vi "ExcimSavePanel.vi"(8 "error in":errorcluster) -> (0 "error out":errorcluster, 3 "Chaîne":string)   [LabVIEW 2010, in "PhotoLum.lvclass"]
uses:
  PhotoLum.lvclass
panel:
  in  "RepRate":i32=5 caption="Taux Répétition(PPS)" min=0 step=1
  in  "OtherMat":string caption="Matériaux (autres)"
  in  "Matériaux":u16(ring) items=["AlGaAs", "AlN", "AlP", "GaAs", "GaN", "Ge", "InP", "Si", "SiGe", "Autres"]
  in  "unit":u16(ring) caption="Unités\nPre-amp." items=["mA/V", "µA/V", "nA/V", "pA/V"]
  in  "Facteur":u16(ring) caption="Facteur Pre-amp." items=["1", "2", "5", "10", "20", "50", "100", "200", "500"]
  in  "Preamp":u16(ring) caption="Pre-amplificateur" items=["Aucun", "SR570 Current Preamp", "SR560 Voltage Preamp"]
  in  "PLaser":dbl=1000.0 caption="Énergie Laser(mJ)" min=0.0 step=0.1 format="%#.1f"
  in  "Temp":dbl=293.0 caption="Température(°K)" min=0.0 step=0.1 format="%#.1f"
  in  "Annuler":bool
  in  "Save":bool
  in  "Autres":string
  in  "Filtre":u16(ring) caption="Filtre Entrée" items=["Aucun", "CGA 225", "Mauve", "Jaune 495nm", "Vert", "Orange", "Rouge 665nm", "Rouge 850nm", "SI"]
  in  "LN Cooled":bool
  in  "Échantillon":string
  in  "Détecteur":u16(ring) items=["Oriel 70680 with R928"]
  in  "Réseaux":u16(ring) items=["Oriel 33010FL01-080R (400nm)", "Oriel 77234 (1um)"]
  in  "2xInput":bool
  in  "OutputSlit":dbl caption="Largeur de fente de sortie (mm)"
  in  "InputSlit":dbl caption="Largeur de fente d'entrée (mm)"
  # "Paramètres du balayage"
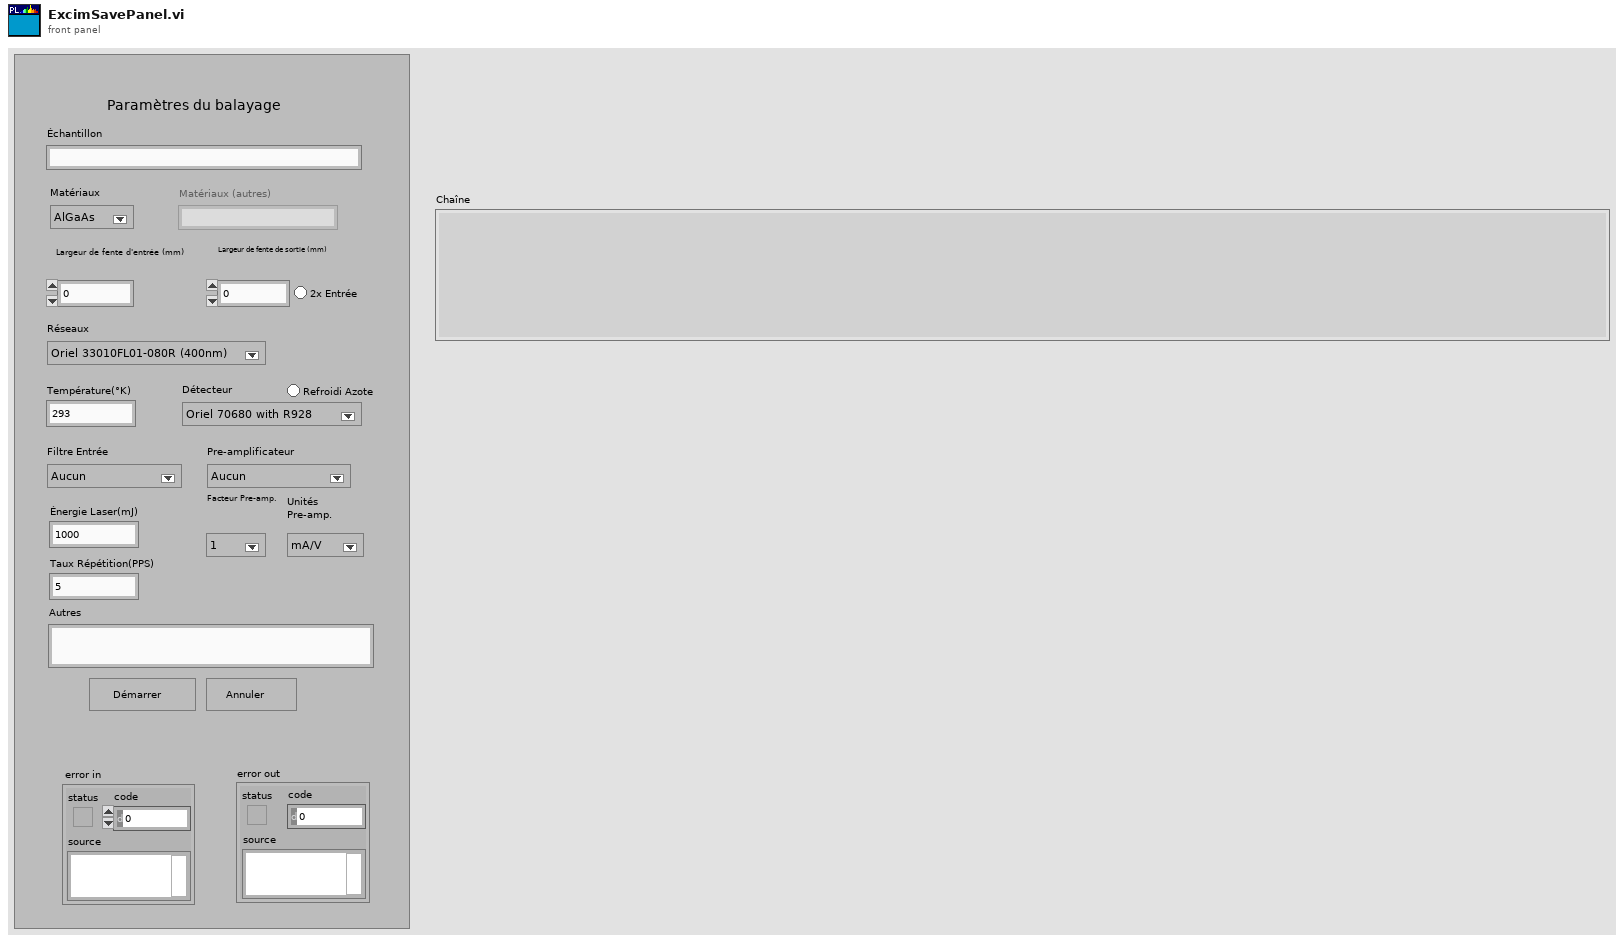
[diagram p1: front panel]
types:
  T1 = enum8{"Enabled", "Disabled", "Disabled and Grayed Out"}
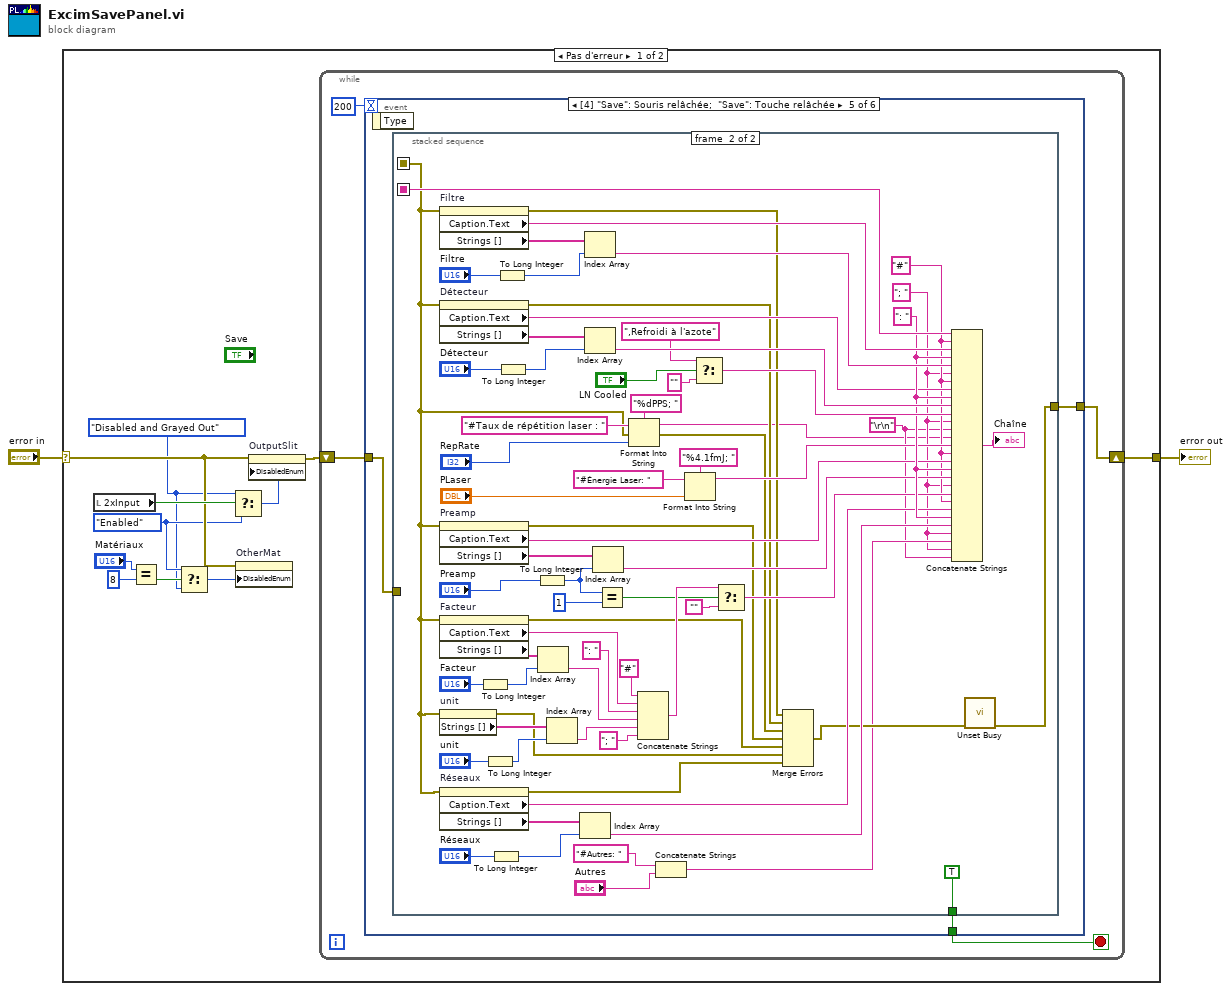
[diagram p0: block diagram]
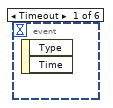
[diagram p2: hidden frame]
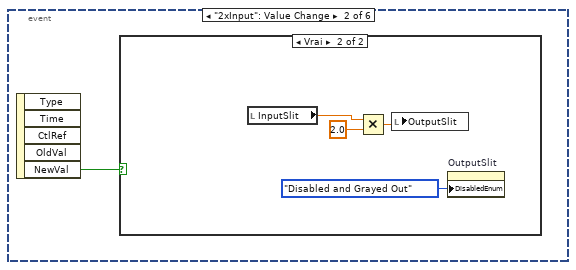
[diagram p3: hidden frame]
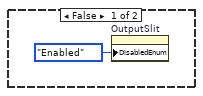
[diagram p4: hidden frame]
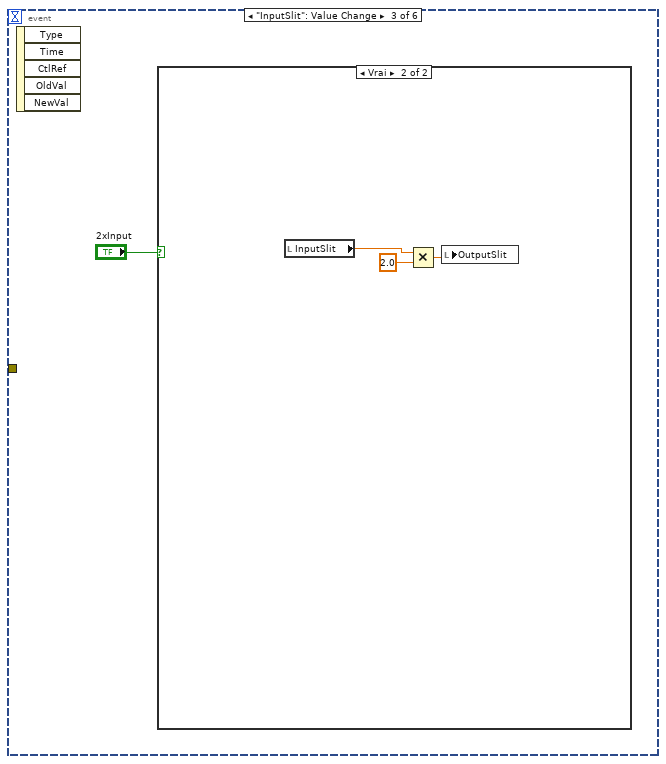
[diagram p5: hidden frame]
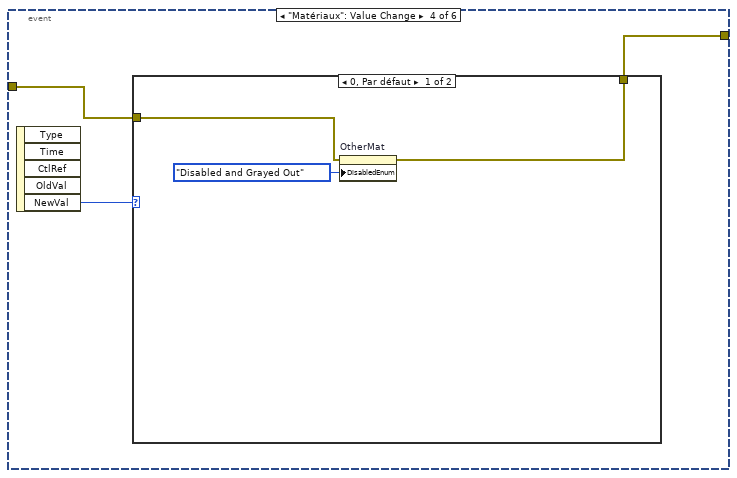
[diagram p7: hidden frame]
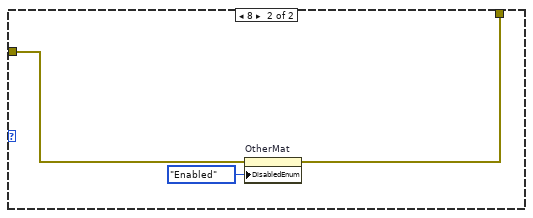
[diagram p8: hidden frame]
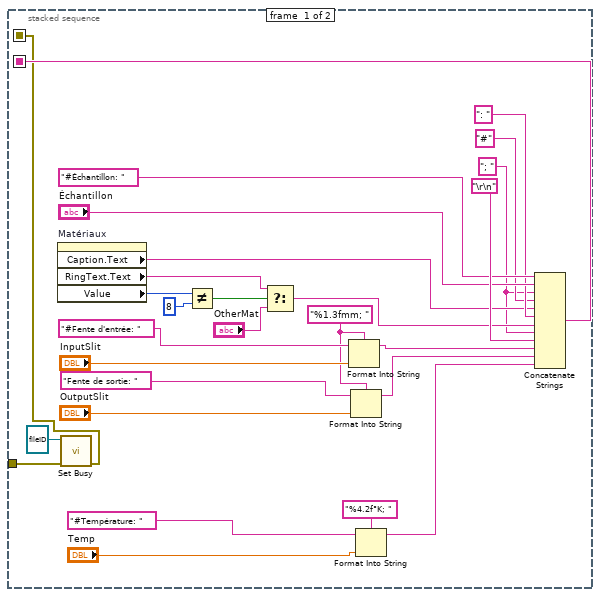
[diagram p9: hidden frame]
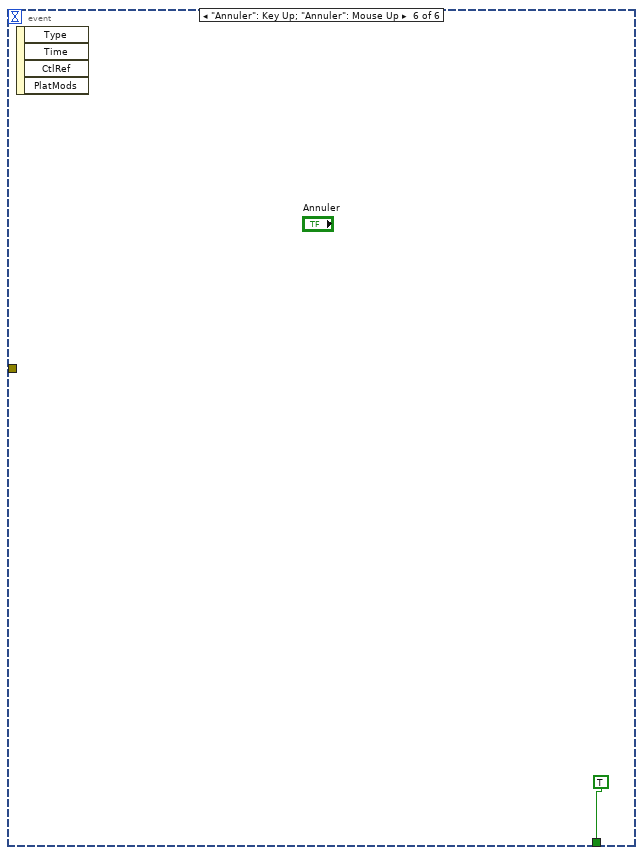
[diagram p10: hidden frame]
diagram:
  n1 = case shown="Pas d'erreur" "error in" {
    selector: "error in" -> [w9 w138]
    tunnel: [w13 w138] -> w2
    frame No Error {
      w4 = T1."Disabled and Grayed Out" ("Désactivé")
      w5 = T1."Enabled" ("Désactivé")
      n2 = local read "2xInput"() -> (w11:bool)
      n3 = Equal?(x="Matériaux", y=u16 8) -> (x = y?=w6:bool)
      n4 = Select(t=w5, s=w6, f=w4) -> (s? t:f=w3:T1)
      n5 = Select(t=w4, s=w11, f=w5) -> (s? t:f=w10:T1)
      n6 = property on="OtherMat" class="Ch"(error in=w9, "DisabledEnum"=w3) -> ()  [unwired: 1 in, 2 out]
      n7 = property on="OutputSlit" class="NumDig (strict)"(error in=w9, "DisabledEnum"=w10) -> (error out=w12:errorcluster)  [unwired: 1 in, 1 out]
      n8 = while {
        shift-right: [w14] -> w13
        shift-left: w12 -> [w15]
        stop <- w16 stop-if-true
        n9 = event shown="[4] \"Save\": Souris relâchée;  \"Save\": Touche relâchée" {
          selector: _ -> [_ _ _ _ _ _]
          dyn-events: _ -> [_ _ _ _ _ _]
          timeout: 200 -> [_ _ _ _ _ _]
          tunnel: [_ _ _ _ w39 TRUE] -> w16
          tunnel: w15 -> [_ _ _ w29 w38 _]
          tunnel: [_ _ _ w28 w37 _] -> w14
          event Timeout {
            n10 = event-data() -> ()  [unwired: 1 in, 2 out]
          }
          event "2xInput": Value Change {
            n11 = event-data() -> ("NewVal"=w18:bool)  [unwired: 1 in, 4 out]
            n12 = case shown="Vrai" w18 {
              frame False {
                n13 = property on="OutputSlit" class="NumDig (strict)"("DisabledEnum"=T1."Enabled" ("Désactivé")) -> ()  [unwired: 2 in, 2 out]
              }
              frame True {
                n14 = local read "InputSlit"() -> (w20:dbl)
                n15 = Multiply(x=w20, y=2.0) -> (x*y=w22:dbl)
                n16 = local write "OutputSlit"(w22) -> ()
                n17 = property on="OutputSlit" class="NumDig (strict)"("DisabledEnum"=T1."Disabled and Grayed Out" ("Désactivé")) -> ()  [unwired: 2 in, 2 out]
              }
            }
          }
          event "InputSlit": Value Change {
            n18 = event-data() -> ()  [unwired: 1 in, 5 out]
            n19 = case shown="Vrai" "2xInput" {
              frame False {
              }
              frame True {
                n20 = local read "InputSlit"() -> (w25:dbl)
                n21 = Multiply(x=w25, y=2.0) -> (x*y=w27:dbl)
                n22 = local write "OutputSlit"(w27) -> ()
              }
            }
          }
          event "Matériaux": Value Change {
            n23 = event-data() -> ("NewVal"=w30:u16)  [unwired: 1 in, 4 out]
            n24 = case shown="0, Par défaut" w30 {
              tunnel: w29 -> [w32 w35]
              tunnel: [w31 w34] -> w28
              frame 0, Default {
                n25 = property on="OtherMat" class="Ch"(error in=w32, "DisabledEnum"=T1."Disabled and Grayed Out" ("Désactivé")) -> (error out=w31:errorcluster)  [unwired: 1 in, 1 out]
              }
              frame 8 {
                n26 = property on="OtherMat" class="Ch"(error in=w35, "DisabledEnum"=T1."Enabled" ("Désactivé")) -> (error out=w34:errorcluster)  [unwired: 1 in, 1 out]
              }
            }
          }
          event "Save": Mouse Up; "Save": Key Up {
            n27 = event-data() -> ()  [unwired: 1 in, 1 out]
            n28 = stacked-sequence {
              seq-local: [w51 _] -> [_ w120]
              seq-local: [w40 _] -> [_ w69]
              tunnel: [_ TRUE] -> w39
              tunnel: w38 -> [w53 _]
              tunnel: [_ w80] -> w37
              frame #0 {
                w58 = "%1.3fmm; " ("chaîne de format")
                w41 = "; " ("chaîne")
                n29 = property on="Matériaux" class="MDér (strict)"() -> ("Caption.Text"=w48:string, "RingText.Text"=w44:string, "Value"=w46:u16)  [unwired: 2 in, 2 out]
                n30 = call <vilib>:"Set Busy.vi"("error in (no error)"=w53, "cursor ID"=refnum<k1> refnum) -> ("error out"=w40:errorcluster)  [unwired: 8 in, 1 out]
                n31 = Not Equal?(x=w46, y=u16 8) -> (x != y?=w45:bool)
                n32 = Select(t=w44, s=w45, f="OtherMat") -> (s? t:f=w42:string)
                n33 = Format Into String(format string=w58, initial string="#Fente d'entrée: " ("chaîne"), "InputSlit") -> (resulting string=w62:string)  [unwired: 1 in, 1 out]
                n34 = Format Into String(format string=w58, initial string="Fente de sortie: " ("chaîne"), "OutputSlit") -> (resulting string=w61:string)  [unwired: 1 in, 1 out]
                n35 = Format Into String(format string="%4.2f°K; " ("chaîne de format"), initial string="#Température: " ("string"), "Temp") -> (resulting string=w54:string)  [unwired: 1 in, 1 out]
                n36 = Concatenate Strings("#Échantillon: " ("chaîne"), "Échantillon", w41, "#" ("string"), w48, ": " ("string"), w42, w41, "\r\n", w62, w61, w54) -> (w51:string)
              }
              frame #1 {
                w87 = "#" ("chaîne")
                w75 = "\r\n"
                w76 = "; " ("chaîne")
                w117 = ": " ("chaîne")
                n37 = property on="Filtre" class="MDér (strict)"(error in=w69) -> (error out=w86:errorcluster, "Caption.Text"=w128:string, "Strings []"=w136:string[])  [unwired: 1 in, 1 out]
                n38 = property on="Détecteur" class="MDér (strict)"(error in=w69) -> (error out=w85:errorcluster, "Caption.Text"=w92:string, "Strings []"=w132:string[])  [unwired: 1 in, 1 out]
                n39 = property on="Preamp" class="MDér (strict)"(error in=w69) -> (error out=w71:errorcluster, "Caption.Text"=w96:string, "Strings []"=w119:string[])  [unwired: 1 in, 1 out]
                n40 = property on="Facteur" class="MDér (strict)"(error in=w69) -> (error out=w84:errorcluster, "Caption.Text"=w100:string, "Strings []"=w107:string[])  [unwired: 1 in, 1 out]
                n41 = property on="unit" class="MDér (strict)"(error in=w69) -> (error out=w82:errorcluster, "Strings []"=w106:string[])  [unwired: 1 in, 1 out]
                n42 = property on="Réseaux" class="MDér (strict)"(error in=w69) -> (error out=w83:errorcluster, "Caption.Text"=w115:string, "Strings []"=w125:string[])  [unwired: 1 in, 1 out]
                n43 = To Long Integer(number="Facteur") -> (32bit integer=w103:i32)
                n44 = To Long Integer(number="unit") -> (32bit integer=w102:i32)
                n45 = To Long Integer(number="Réseaux") -> (32bit integer=w130:i32)
                n46 = To Long Integer(number="Filtre") -> (32bit integer=w134:i32)
                n47 = To Long Integer(number="Détecteur") -> (32bit integer=w133:i32)
                n48 = To Long Integer(number="Preamp") -> (32bit integer=w111:i32)
                n49 = Index Array(array=w107, index=w103) -> (element=w98:string)
                n50 = Index Array(array=w106, index=w102) -> (element=w101:string)
                n51 = Index Array(array=w125, index=w130) -> (element=w93:string)
                n52 = Index Array(array=w136, index=w134) -> (element=w127:string)
                n53 = Index Array(array=w132, index=w133) -> (element=w126:string)
                n54 = Index Array(array=w119, index=w111) -> (element=w116:string)
                n55 = Equal?(x=w111, y=1) -> (x = y?=w94:bool)
                n56 = Format Into String(format string="%dPPS; " ("chaîne de format"), initial string="#Taux de répétition laser : " ("string"), error in=w69, "RepRate") -> (resulting string=w68:string, error out=w70:errorcluster)
                n57 = Concatenate Strings("#" ("chaîne"), w100, ": " ("chaîne"), w98, w101, "; " ("chaîne")) -> (w95:string)
                n58 = Concatenate Strings("#Autres: " ("chaîne"), "Autres") -> (w77:string)
                n59 = Format Into String(format string="%4.1fmJ; " ("chaîne de format"), initial string="#Énergie Laser: " ("string"), "PLaser") -> (resulting string=w112:string)  [unwired: 1 in, 1 out]
                n60 = Select(t=",Refroidi à l'azote" ("chaîne"), s="LN Cooled", f="" ("chaîne")) -> (s? t:f=w121:string)
                n61 = Select(t=w95, s=w94, f="") -> (s? t:f=w108:string)
                n62 = Merge Errors(w86, w85, w70, w71, w84, w82, w83) -> (w81:errorcluster)
                n63 = Concatenate Strings(w120, w87, w128, w117, w127, w76, w87, w92, w117, w126, w121, w76, w75, w68, w112, w87, w96, w117, w116, w76, w108, w87, w115, w117, w93, w76, w77, w76, w75) -> (→"Chaîne":string)
                n64 = call <vilib>:"Unset Busy.vi"("error in (no error)"=w81) -> ("error out"=w80:errorcluster)  [unwired: 10 in]
              }
            }
          }
          event "Annuler": Key Up; "Annuler": Mouse Up {
            n65 = event-data() -> ()  [unwired: 1 in, 4 out]
          }
        }
      }
    }
    frame Error {
    }
  }
  "error out" <- w2
